vi "WorkorderHandler_GetActScriptOrder.vi"(8 "error in (no error)":errorcluster, 11 "reference":T1) -> (0 "error out":errorcluster, 1 "Order":string, 2 "Script":string, 3 "duplicate reference":T1)   [LabVIEW 2011]
uses:
  DataStructures/WorkorderHandler_ObjectReference.ctl
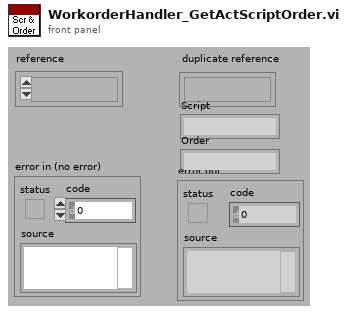
[diagram p1: front panel]
types:
  T1 = typedef "WorkorderHandler_ObjectReference.ctl" = refnum<k1>
  T2 = typedef "WorkorderHandler_ObjectData.ctl" = cluster{"Table":string[][], "Script":string, "Order":string, "No":string, "Time":dbl}
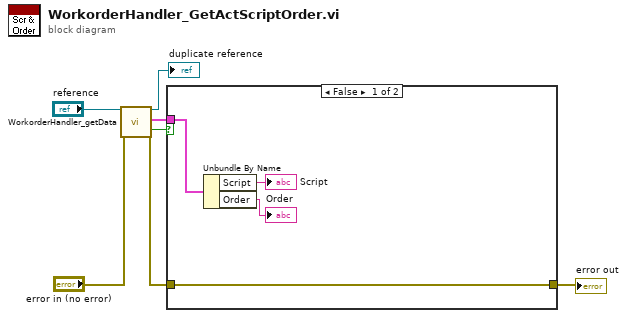
[diagram p0: block diagram]
diagram:
  n1 = call "WorkorderHandler_getData.vi"("reference"="reference", "error in (no error)"="error in (no error)") -> ("duplicate reference"=→"duplicate reference":T1, "data"=w5:T2, "timed out?"=w1:bool, "error out"=w2:errorcluster)  [unwired: 1 in, 13 out]
  n2 = case shown="False" w1 {
    tunnel: w5 -> [w11 _]
    tunnel: [w10 w12] -> w4
    tunnel: w2 -> [w10 w12]
    frame False {
      n3 = Unbundle By Name(w11) -> ("Script"=→"Script":string, "Order"=→"Order":string)
    }
    frame True {
      # "Error or Timed Out"
    }
  }
  "error out" <- w4
